vi "Index 1D Array Elements (Boolean)__ogtk.vi"(9 "indices":i32[](array[numeric]), 11 "array":bool[](array[boolean])) -> (1 "elements":bool[](array[boolean]))   [LabVIEW 2020]
doc: "This polymorphic VI returns the <B>elements</B> of a 1D or 2D <B>array</B> at the corresponding <B>indices</B>. For 2D arrays, wire both the <B>indices 0</B> and <B>indices 1</B> inputs to specify the desired <B>elements</B>."
panel:
  # "Index Array Elements.vi\n\nReturns the elements of an array at the corresponding indices.\n\nPlease visit http://www.OpenG.org to learn about the\nOpen Source LabVIEW software movement.\n\nNOTICE -- YOU MUST LEAVE THIS NOTICE IN PLACE.  PER THE TERMS OF THE LICENSE BELOW, YOU MAY SUBLICENSE THIS SOFTWARE \nIN ANY WAY THAT DOES NOT CONFLICT WITH THIS LICENSE.\n\n### BSD License (http://www.opensource.org/licenses/bsd-license.php) Begin ###\n \nCopyright (c) 2007, JKI <info@jameskring.com> (Author: Jim Kring <jim.kring@jameskring.com>)\n\nAll rights reserved.\n\nRedistribution and use in source and binary forms, with or without modification, are permitted provided that the following conditions are met:\n\n    * Redistributions of source code must retain the above copyright notice, this list of conditions and the following disclaimer.\n    * Redistributions in binary form must reproduce the above copyright notice, this list of conditions and the following disclaimer in the \n       documentation and/or other materials provided with the distribution.\n    * Neither the name of SciWare, James Kring, Inc., nor the names of its contributors may be used to endorse or promote products derived \n       from this software without specific prior written permission.\n\nTHIS SOFTWARE IS PROVIDED BY THE COPYRIGHT HOLDERS AND CONTRIBUTORS \"AS IS\" AND ANY EXPRESS OR IMPLIED WARRANTIES, \nINCLUDING, BUT NOT LIMITED TO, THE IMPLIED WARRANTIES OF MERCHANTABILITY AND FITNESS FOR A PARTICULAR PURPOSE ARE \nDISCLAIMED. IN NO EVENT SHALL THE COPYRIGHT OWNER OR CONTRIBUTORS BE LIABLE FOR ANY DIRECT, INDIRECT, INCIDENTAL,\n SPECIAL, EXEMPLARY, OR CONSEQUENTIAL DAMAGES (INCLUDING, BUT NOT LIMITED TO, PROCUREMENT OF SUBSTITUTE GOODS OR \nSERVICES; LOSS OF USE, DATA, OR PROFITS; OR BUSINESS INTERRUPTION) HOWEVER CAUSED AND ON ANY THEORY OF LIABILITY, \nWHETHER IN CONTRACT, STRICT LIABILITY, OR TORT (INCLUDING NEGLIGENCE OR OTHERWISE) ARISING IN ANY WAY OUT OF THE USE \nOF THIS SOFTWARE, EVEN IF ADVISED OF THE POSSIBILITY OF SUCH DAMAGE.\n\n### BSD License End ###"
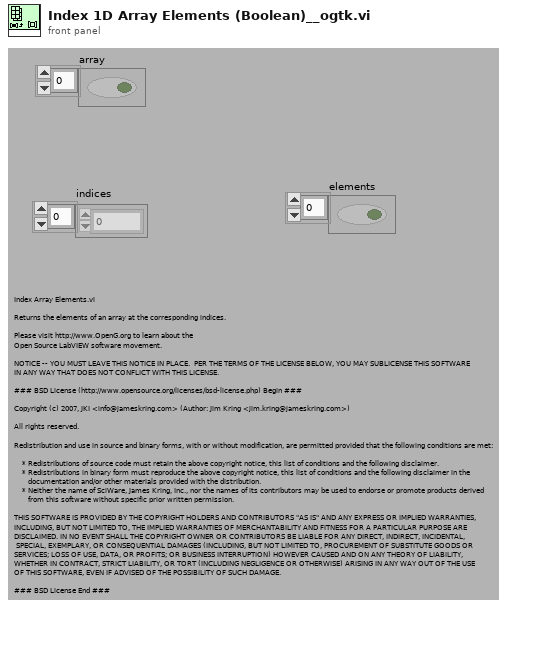
[diagram p1: front panel]
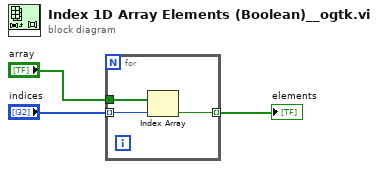
[diagram p0: block diagram]
diagram:
  n1 = for {
    tunnel: "indices" -> [w6] mode=indexing
    tunnel: "array" -> [w5]
    tunnel: [w4] -> w1 mode=indexing
    n2 = Index Array(array=w5, index=w6) -> (element=w4:bool)
  }
  "elements" <- w1
